vi "RadialProfileToImage.vi"(6 "Center y":dbl, 8 "Center x":dbl, 9 "Width":dbl, 10 "Height":dbl, 11 "Radial counts":dbl[](array[numeric])) -> (3 "Output":dbl[][](array[numeric]))   [LabVIEW 2010]
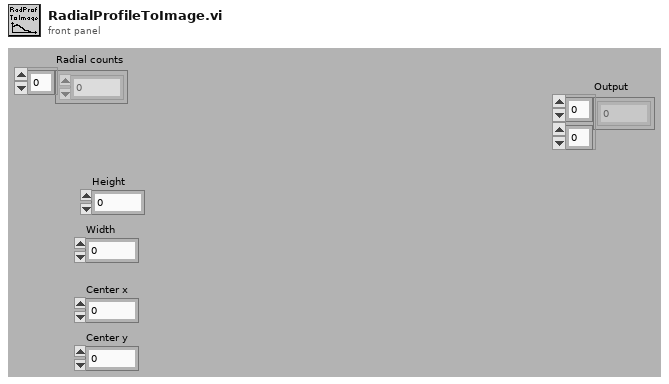
[diagram p1: front panel]
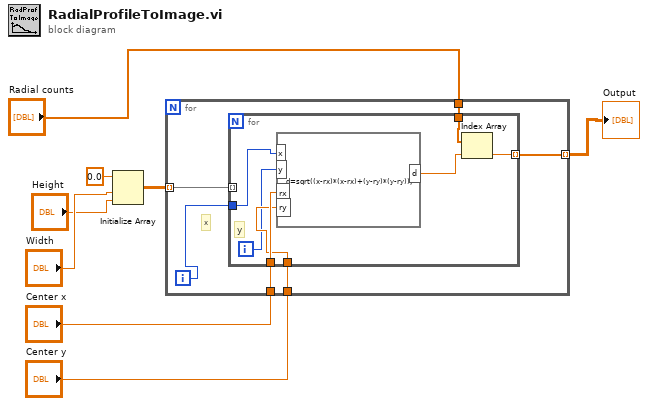
[diagram p0: block diagram]
diagram:
  n1 = Initialize Array(0.0 ("element"), "Width", "Height") -> (w5:dbl[][])
  n2 = for {
    tunnel: w5 -> [w14] mode=indexing
    tunnel: "Center x" -> [w12]
    tunnel: "Center y" -> [w11]
    tunnel: "Radial counts" -> [w10]
    tunnel: [w9] -> w1 mode=indexing
    i -> [w13]
    # "x"
    n3 = for {
      tunnel: w14 -> [_] mode=indexing
      tunnel: w13 -> [w19]
      tunnel: w12 -> [w21]
      tunnel: w11 -> [w20]
      tunnel: w10 -> [w17]
      tunnel: [w15] -> w9 mode=indexing
      i -> [w18]
      # "y"
      n4 = formula code="d=sqrt((x-rx)*(x-rx)+(y-ry)*(y-ry));"("x"=w19, "y"=w18, "rx"=w21, "ry"=w20) -> ("d"=w16:dbl)
      n5 = Index Array(array=w17, index=w16) -> (element=w15:dbl)
    }
  }
  "Output" <- w1
